vi "CheckExposure.vi"(6 "error constant":errorcluster, 8 "Sensor readout time":dbl format="%#_13g", 9 "Frame Rate":dbl, 10 "Exposure Time":dbl, 11 "Exposure Start Delay":dbl) -> (0 "error out":errorcluster)   [LabVIEW 2023]
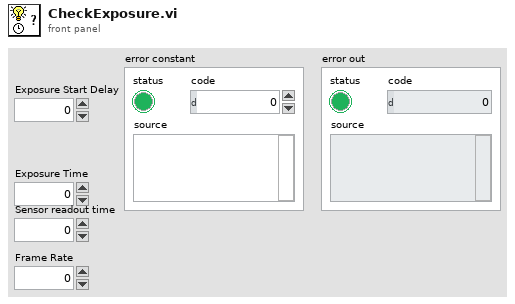
[diagram p1: front panel]
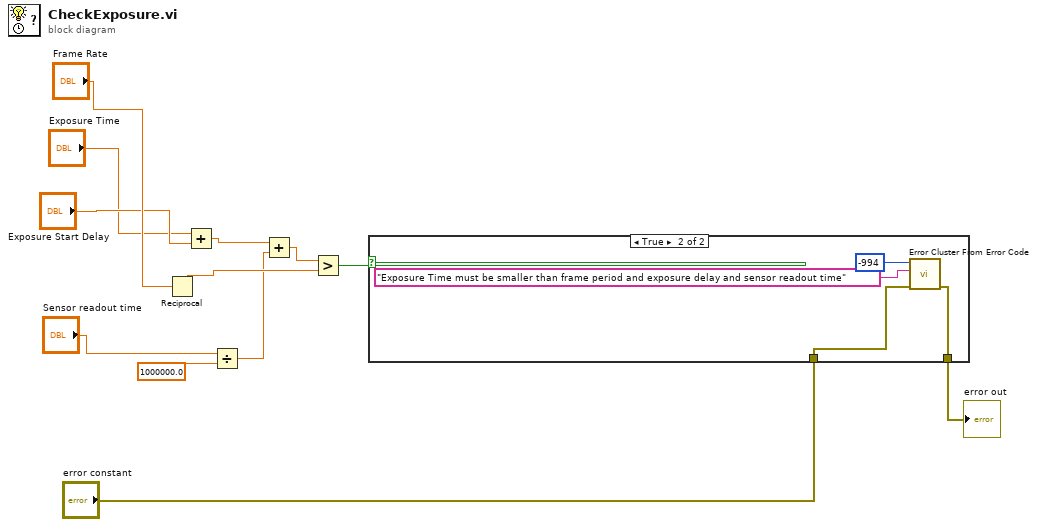
[diagram p0: block diagram]
diagram:
  n1 = Reciprocal(x="Frame Rate") -> (1/x=w10:dbl)
  n2 = Add(x="Exposure Time", y="Exposure Start Delay") -> (x+y=w7:dbl)
  n3 = Divide(x="Sensor readout time", y=1000000.0) -> (x/y=w3:dbl)
  n4 = Add(x=w7, y=w3) -> (x+y=w6:dbl)
  n5 = Greater?(x=w6, y=w10) -> (0:w12:bool)
  n6 = case shown="True" w12 {
    tunnel: [w13 w15] -> w5
    tunnel: "error constant" -> [w13 w14]
    frame False {
    }
    frame True {
      n7 = call <vilib>:"Error Cluster From Error Code.vi"("error in (no error)"=w14, "error message (\"\")"="Exposure Time must be smaller than frame period and exposure delay and sensor readout time" ("error message (\"\")"), "error code (0)"=-994) -> ("error out"=w15:errorcluster)  [unwired: 6 in]
    }
  }
  "error out" <- w5
